vi "setSettingsVert.vi"(7 "Active Channel":string, 8 "error out in":errorcluster, 10 "Channel settings":T1, 11 "IVI Refnum in":refnum<k15>) -> (0 "error out out":errorcluster, 2 "Channel settings out":T1, 3 "IVI Refnum out":refnum<k15>)   [LabVIEW 2011]
uses:
  ChannelSettings_TypDef.ctl
  coupling_Enum_TypDef.ctl
  impedance_Enum_TypDEf.ctl
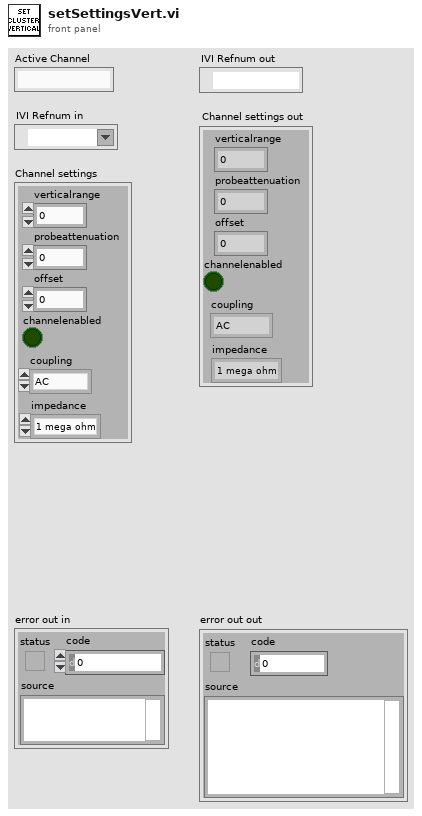
[diagram p1: front panel]
types:
  T1 = typedef "ChannelSettings_TypDef.ctl" = cluster{"verticalrange":dbl, "probeattenuation":dbl, "offset":dbl, "channelenabled":bool, "coupling":T2, "impedance":T3}
  T2 = typedef "coupling_Enum_TypDef.ctl" = enum16{"AC", "DC", "Ground"}
  T3 = typedef "impedance_Enum_TypDEf.ctl" = enum16{"1 mega ohm", "<NA>", "50 ohms"}
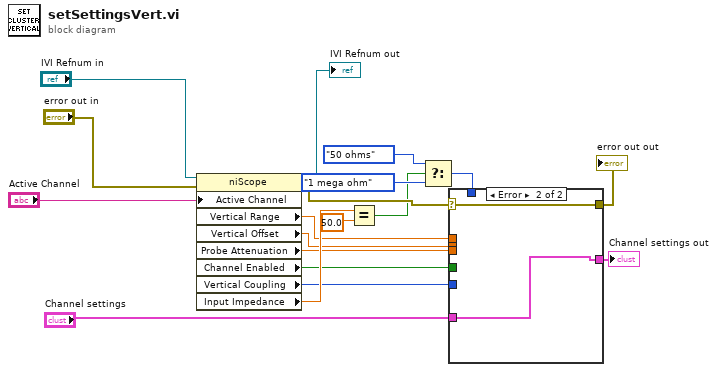
[diagram p0: block diagram]
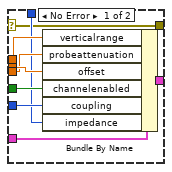
[diagram p2: hidden frame]
diagram:
  n1 = property class="niScope"(reference="IVI Refnum in", error in="error out in", "Active Channel"="Active Channel") -> (reference out=→"IVI Refnum out":refnum<k15>, error out=w19:errorcluster, "Vertical Range"=w4:dbl, "Vertical Offset"=w5:dbl, "Probe Attenuation"=w6:dbl, "Channel Enabled"=w7:bool, "Vertical Coupling"=w8:i32, "Input Impedance"=w10:dbl)
  n2 = Equal?(x=w10, y=50.0) -> (x = y?=w12:bool)
  n3 = Select(t=impedance_Enum_TypDEf."50 ohms" ("impedance"), s=w12, f=impedance_Enum_TypDEf."1 mega ohm" ("impedance")) -> (s? t:f=w13:T3)
  n4 = case shown="Error" w19 {
    selector: w19 -> [w20 w29]
    tunnel: [w28 w30] -> w3
    tunnel: w4 -> [w27 _]
    tunnel: w5 -> [w26 _]
    tunnel: w6 -> [w25 _]
    tunnel: w7 -> [w24 _]
    tunnel: w8 -> [w23 _]
    tunnel: w13 -> [w22 _]
    tunnel: "Channel settings" -> [w21 w30]
    tunnel: [w20 w29] -> w1
    frame No Error {
      n5 = Bundle By Name(cluster=w21, "verticalrange"=w27, "probeattenuation"=w25, "offset"=w26, "channelenabled"=w24, "coupling"=w23, "impedance"=w22) -> (w28:T1)
    }
    frame Error {
    }
  }
  "Channel settings out" <- w3
  "error out out" <- w1
